vi "Open Image.vi"(5 "prompt":string="Select an image view", 7 "start path  (Not A Path)":path=path "", 8 "error in (no error)":errorcluster, 11 "Image":T1) -> (0 "error out":errorcluster, 2 "Image Out":T1, 3 "Image opened?":bool)   [LabVIEW 2013, in "FileIO lib.lvlib"]
doc: "Opens the image from the specified path and puts it into the incoming image space."
uses:
  FileIO lib.lvlib
  <vilib>/vision/Image Controls.llb/IMAQ Image.ctl
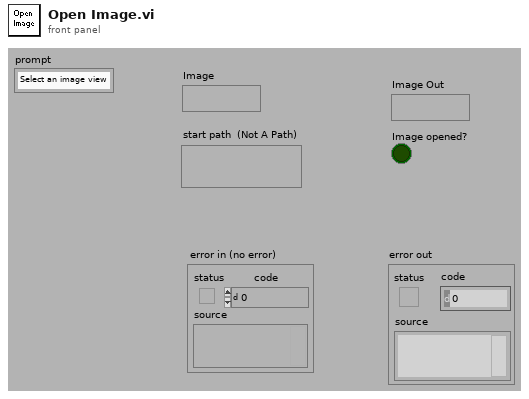
[diagram p1: front panel]
types:
  T1 = typedef "IMAQ Image.ctl" = refnum<image>
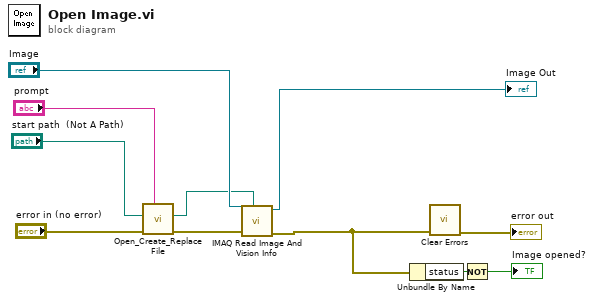
[diagram p0: block diagram]
diagram:
  n1 = call <vilib>:"Open_Create_Replace File.vi"("prompt"="prompt", "error in (no error)"="error in (no error)", "start path  (Not A Path)"="start path  (Not A Path)") -> ("error out"=w2:errorcluster, "new file path"=w3:path)  [unwired: 3 in, 4 out]
  n2 = call "IMAQ Read Image And Vision Info"("File Path"=w3, "error in (no error)"=w2, "Image"="Image") -> ("error out"=w1:errorcluster, "Image Out"=→"Image Out":T1)  [unwired: 6 in, 1 out]
  n3 = Unbundle By Name(w1) -> ("status"=w8:bool)
  n4 = call <vilib>:"Clear Errors.vi"("error in (no error)"=w1) -> ("error out"=→"error out":errorcluster)  [unwired: 6 out]
  n5 = Not(x=w8) -> (.not. x?=→"Image opened?":bool)
